vi "WPI_DriverStationReport Robot Code State.vi"(7 "Test":bool, 8 "error in (no error)":errorcluster, 9 "TeleOp":bool, 10 "Autonomous":bool, 11 "Disabled":bool) -> (0 "error out":errorcluster)   [LabVIEW 2017]
doc: "Reports whether the robot code is running in Disabled, Autonomous, Teleop, or Test mode. Use the <B>Charts</B> page of the FRC Driver Station or the FRC DS Log File Viewer to track what code actually runs and how often it runs to ensure the code runs as you intend."
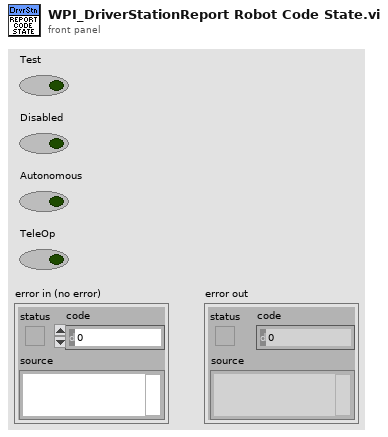
[diagram p1: front panel]
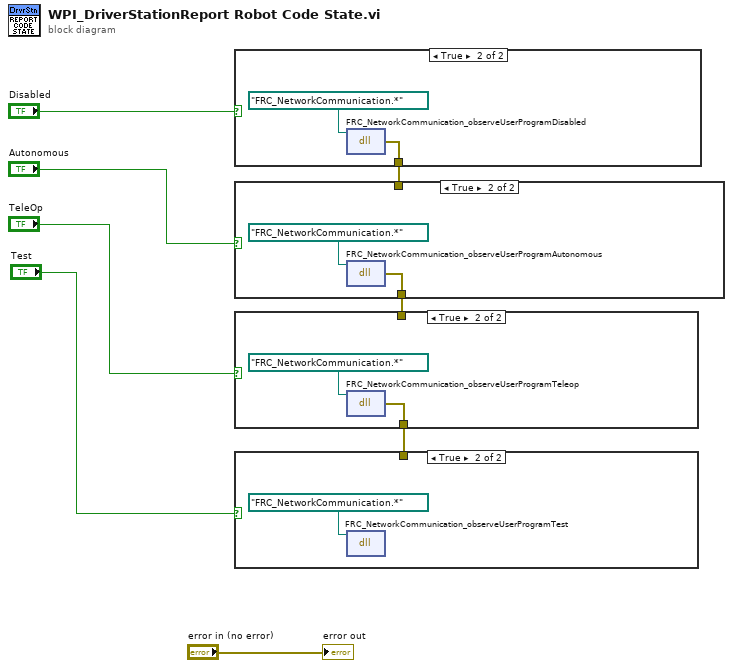
[diagram p0: block diagram]
diagram:
  n1 = case shown="True" "Disabled" {
    tunnel: [_ w9] -> w3
    frame False {
    }
    frame True {
      n2 = dll-call lib="?" fn="FRC_NetworkCommunication_observeUserProgramDisabled"(path in=path "FRC_NetworkCommunication.*") -> (error out=w9:errorcluster)  [unwired: 2 in, 2 out]
    }
  }
  n3 = case shown="True" "Autonomous" {
    tunnel: w3 -> [_ _]
    tunnel: [_ w11] -> w2
    frame False {
    }
    frame True {
      n4 = dll-call lib="?" fn="FRC_NetworkCommunication_observeUserProgramAutonomous"(path in=path "FRC_NetworkCommunication.*") -> (error out=w11:errorcluster)  [unwired: 2 in, 2 out]
    }
  }
  n5 = case shown="True" "TeleOp" {
    tunnel: w2 -> [_ _]
    tunnel: [_ w13] -> w1
    frame False {
    }
    frame True {
      n6 = dll-call lib="?" fn="FRC_NetworkCommunication_observeUserProgramTeleop"(path in=path "FRC_NetworkCommunication.*") -> (error out=w13:errorcluster)  [unwired: 2 in, 2 out]
    }
  }
  n7 = case shown="True" "Test" {
    tunnel: w1 -> [_ _]
    frame False {
    }
    frame True {
      n8 = dll-call lib="?" fn="FRC_NetworkCommunication_observeUserProgramTest"(path in=path "FRC_NetworkCommunication.*") -> ()  [unwired: 2 in, 3 out]
    }
  }
  "error out" <- "error in (no error)"
